vi "Gyro (SubVI).vi"   [LabVIEW 2016]
uses:
  <vilib>/Rock Robotics/Network Tables/SD Write Number.vi
types:
  T1 = typedef "WPI_GyroDevRef.ctl" = cluster{"DevStatus":errorcluster, "Analog Channel":T2, "Offset":dbl, "Gain (VoltsPerDegree/Second)":dbl, "Gyro Type":enum16{"Analog", "XRS450"}, "Handle":i32, "SPI Bus":T3, "Device Found":bool, "Sample Rate":dbl, "Calibrate On Open":bool}
  T2 = typedef "FPGA_AIChannel.ctl" = enum8{"AI 0", "AI 1", "AI 2", "AI 3", "AI MXP 0", "AI MXP 1", "AI MXP 2", "AI MXP 3", "Invalid"}
  T3 = typedef "spi_bus.ctl" = enum16{"SPI On-Board, CS0", "SPI On-Board, CS1", "SPI On-Board, CS2", "SPI On-Board, CS3", "SPI MXP", "Invalid"}
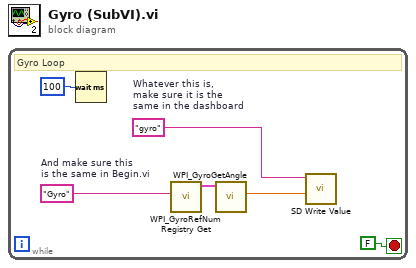
[diagram p0: block diagram]
diagram:
  n1 = while {
    stop <- FALSE stop-if-true
    w2 = "Gyro"  # And make sure this is the same in Begin.vi
    w4 = "gyro"  # Whatever this is,  make sure it is the  same in the dashboard
    # "Gyro Loop"
    n2 = Wait (ms)(milliseconds to wait=u32 100) -> ()  [unwired: 1 out]
    n3 = call <vilib>:"WPI_GyroRefNum Registry Get.vi"("refnum name"=w2) -> ("GyroDevRef"=w3:T1)  [unwired: 9 in, 1 out]
    n4 = call <vilib>:"WPI_GyroGetAngle.vi"("GyroDevRef"=w3) -> ("Angle"=w1:dbl)  [unwired: 7 in, 3 out]
    n5 = call-poly <vilib>:"SD Write Value.vi"("Numeric"=w1, "Name"=w4) -> ()  [unwired: 8 in, 2 out]
  }
